vi "BenchA_v09_979.vi"() -> ()   [LabVIEW 2017]
uses:
  x64/Debug/BERTTA.dll
panel:
  out "element":bool
  out "Started:":string
  in  "SHUTDOWN":bool
  in  "MASTER CONTROL":bool
  in  "Tab Control":T1(tab)
  out "Output File":path caption="selected path"
  in  "Browse folder":path=path "" caption="start path"
  in  "Read Seq":bool
  in  "Save Seq":bool
  in  "Configuration file":path=path "C:/Users/shresplab/Desktop/BerttaConfiguration.lvm" caption="Filename"
  in  "OK Button 2":bool
  out "Boolean":bool
  in  "User (initials)":string
  in  "Project name":string
  in  "Description":string
  out "PUMP1":bool
  out "Target amount":dbl
  out "Scale weight":dbl
  out "Amount now":dbl
  out "Flow rate":dbl
  out "Time to target":dbl format="%<%H:%M:%S>t"
  out "Current step":dbl
  out "Target":dbl
  out "Amount now":dbl
  out "Amount now":dbl
  out "Target":dbl
  out "Current step":dbl
  out "Time to target":dbl format="%<%H:%M:%S>t"
  out "Flow rate":dbl
  out "Amount now":dbl
  out "Scale weight":dbl
  out "Target amount":dbl
  out "PUMP2":bool
  out "Sensor OK 6":bool
  out "Sensor OK 5":bool
  out "Sensor OK 4":bool
  out "Sensor OK 3":bool
  in  "OK Button":bool
  in  "Add comment":string
  out "PUMP3":bool
  out "Target amount":dbl
  out "Scale weight":dbl
  out "Amount now":dbl
  out "Flow rate":dbl
  out "Time to target":dbl format="%<%H:%M:%S>t"
  out "Current step":dbl
  out "Target":dbl
  out "Amount now":dbl
  out "Tr":dbl
  out "Tj in":dbl
  out "Tj out":dbl
  out "T set":dbl
  out "Current step":i32
  out "RPM":dbl
  out "Torque 2":dbl
  out "Waveform Chart 5":dynamicdata(graph)
  out "Waveform Chart 6":dynamicdata(graph)
  out "Waveform Chart 7":dynamicdata(graph)
  in  "Tab Control 2":T2(tab)
  out "Waveform Chart 3":dynamicdata(graph)
  out "Waveform Chart 8":dynamicdata(graph)
  out "Waveform Chart 11":dynamicdata(graph)
  out "Waveform Chart 13":dynamicdata(graph)
  out "Waveform Chart 9":dynamicdata(graph)
  out "Table":string[][](table)=[["14.8.2017 18.06.59", "0,000000", "417,670000", "-0,150000", "1,000000", "22,220000", "23,366837", "23,574959", "23,985852", "23,690000", "240,000000", "4,000000", "0,000000", "397,000000", "-397,000000", "1,000000"], ["14.8.2017 18.07.06", "0,000000", "417,640000", "-0,120000", "1,000000", "22,220000", "23,763115", "23,906257", "23,985694", "23,680000", "240,000000", "4,000000", "0,000000", "397,000000", "-397,000000", "1,000000"], ["14.8.2017 18.07.13", "0,000000", "417,640000", "-0,120000", "1,000000", "22,220000", "23,965922", "24,013440", "23,984906", "23,670000", "240,000000", "4,100000", "3,000000", "397,000000", "-397,000000", "1,000000"], ["14.8.2017 18.07.21", "0,000000", "417,640000", "-0,120000", "1,000000", "22,220000", "23,943860", "23,900110", "23,987113", "23,670000", "240,000000", "4,000000", "0,000000", "397,000000", "-397,000000", "1,000000"], ["14.8.2017 18.07.28", "0,000000", "417,640000", "-0,120000", "1,000000", "22,220000", "23,736328", "23,600018", "23,989004", "23,660000", "240,000000", "4,000000", "0,000000", "397,000000", "-397,000000", "1,000000"], ["14.8.2017 18.07.36", "0,000000", "417,640000", "-0,120000", "1,000000", "22,220000", "23,480910", "23,324538", "23,991053", "23,660000", "240,000000", "4,000000", "0,000000", "397,000000", "-397,000000", "1,000000"], ["14.8.2017 18.07.43", "0,000000", "417,640000", "-0,120000", "2,000000", "22,220000", "23,195579", "23,008270", "23,999093", "23,650000", "240,000000", "4,000000", "0,000000", "397,000000", "-397,000000", "1,000000"], ["14.8.2017 18.07.51", "0,000000", "417,650000", "-417,650000", "1,000000", "22,220000", "22,862541", "22,649021", "24,003979", "23,650000", "240,000000", "4,000000", "0,000000", "397,000000", "-397,000000", "2,000000"], ["14.8.2017 18.07.58", "0,000000", "417,640000", "0,010000", "1,000000", "22,220000", "22,541353", "22,354878", "24,005398", "23,650000", "240,000000", "4,000000", "0,000000", "397,000000", "-397,000000", "1,000000"], ["14.8.2017 18.08.06", "0,000000", "417,640000", "0,010000", "1,000000", "22,220000", "22,347931", "22,253738", "24,007605", "23,640000", "240,000000", "4,100000", "0,000000", "397,000000", "-397,000000", "1,000000"], ["14.8.2017 18.08.13", "0,000000", "417,640000", "0,010000", "1,000000", "22,220000", "22,329030", "22,302102", "24,006028", "23,640000", "240,000000", "4,000000", "0,000000", "395,820000", "-395,820000", "1,000000"], ["14.8.2017 18.08.20", "0,000000", "417,640000", "0,010000", "1,000000", "22,220000", "22,466849", "22,511320", "24,002403", "23,630000", "240,000000", "4,000000", "0,000000", "395,830000", "-0,010000", "1,000000"], ["14.8.2017 18.08.28", "0,000000", "417,640000", "0,010000", "1,000000", "22,220000", "22,707062", "22,835101", "24,000984", "23,620000", "240,000000", "4,000000", "0,000000", "395,830000", "-0,010000", "1,000000"], ["14.8.2017 18.08.35", "0,000000", "417,640000", "0,010000", "1,000000", "22,220000", "23,054104", "23,232979", "24,001299", "23,600000", "240,000000", "4,000000", "0,000000", "395,830000", "-0,010000", "1,000000"], ["14.8.2017 18.08.43", "0,000000", "417,640000", "0,010000", "1,000000", "22,220000", "23,412371", "23,522793", "24,002560", "23,590000", "240,000000", "4,000000", "0,000000", "395,820000", "0,000000", "1,000000"], ["14.8.2017 18.08.51", "0,000000", "417,640000", "0,010000", "1,000000", "22,220000", "23,596247", "23,656125", "24,003821", "23,580000", "240,000000", "4,000000", "0,000000", "395,820000", "0,000000", "1,000000"]]
  out "Boolean 4":bool
  out "Boolean 3":bool
  out "Boolean 2":bool
  in  "Reset 6":bool
  in  "Manual/Ramp":bool=TRUE
  in  "Array":dbl[][](array[numeric])=[[20.0, 0.0], [20.0, 0.0], [20.0, 0.0]]
  in  "?":bool
  in  "Time":dbl format="Time to target (min):                %#_g"
  out "Current temp":dbl format="Current temperature (S1):   %#_6g"
  in  "OK Button 3":bool
  in  "T ext / T ext 2":enum32{"Sensor 1", "Sensor 2"}(radio)
  out "Sensor OK":bool
  in  "T fail":dbl=20.0 format="Failsafe temperature:              %#_g"
  in  "Setpoint":dbl=20.0 format="Temperature target:                %#_6g"
  in  "Manual select":T3(radio)
  out "Waveform Chart":dynamicdata(graph)
  out "T external 2":dbl format="Current temperature (S2):    %#_g"
  in  "UPDATE TEMP":bool
  out "Led11 5":bool
  out "RPM":dbl format="%_4f"
  out "Led10 3":bool
  out "Led9 3":bool
  out "Led8 3":bool
  out "Led7 3":bool
  out "Led6 3":bool
  out "Led5 3":bool
  out "Led4 3":bool
  out "Led3 3":bool
  out "Led2 3":bool
  out "Led1 3":bool
  in  "PumpSeq 4":dbl[][](array[numeric])=[[0.0, 0.0, 0.0, 0.0, 0.0, 0.0, 0.0, 0.0, 0.0, 0.0], [0.0, 0.0, 0.0, 0.0, 0.0, 0.0, 0.0, 0.0, 0.0, 0.0], [0.0, 0.0, 0.0, 0.0, 0.0, 0.0, 0.0, 0.0, 0.0, 0.0], [0.0, 0.0, 0.0, 0.0, 0.0, 0.0, 0.0, 0.0, 0.0, 0.0], [0.0, 0.0, 0.0, 0.0, 0.0, 0.0, 0.0, 0.0, 0.0, 0.0], [0.0, 0.0, 0.0, 0.0, 0.0, 0.0, 0.0, 0.0, 0.0, 0.0], [0.0, 0.0, 0.0, 0.0, 0.0, 0.0, 0.0, 0.0, 0.0, 0.0], [0.0, 0.0, 0.0, 0.0, 0.0, 0.0, 0.0, 0.0, 0.0, 0.0], [0.0, 0.0, 0.0, 0.0, 0.0, 0.0, 0.0, 0.0, 0.0, 0.0], [0.0, 0.0, 0.0, 0.0, 0.0, 0.0, 0.0, 0.0, 0.0, 0.0]]
  in  "?":bool
  out "Flow rate (g/min)":dbl
  out "Scale reading":dbl
  out "Step amount now":dbl
  in  "Grams / min":dbl
  out "Waveform Chart 14":dynamicdata(graph)
  in  "?":bool
  out "Total amount now":dbl
  out "Led11 4":bool
  in  "Reset 5":bool
  out "Elapsed / step":i32
  out "Time to target":dbl format="%<%H:%M:%S>t"
  in  "OK Button 4":bool
  out "Led11":bool
  out "RPM":dbl format="%_4f"
  out "Led10":bool
  out "Led9":bool
  out "Led8":bool
  out "Led7":bool
  out "Led6":bool
  out "Led5":bool
  out "Led4":bool
  out "Led3":bool
  out "Led2":bool
  out "Led1":bool
  in  "PumpSeq 2":dbl[][](array[numeric])=[[0.0, 0.0, 0.0, 0.0, 0.0, 0.0, 0.0, 0.0, 0.0, 0.0], [0.0, 0.0, 0.0, 0.0, 0.0, 0.0, 0.0, 0.0, 0.0, 0.0], [0.0, 0.0, 0.0, 0.0, 0.0, 0.0, 0.0, 0.0, 0.0, 0.0], [0.0, 0.0, 0.0, 0.0, 0.0, 0.0, 0.0, 0.0, 0.0, 0.0], [0.0, 0.0, 0.0, 0.0, 0.0, 0.0, 0.0, 0.0, 0.0, 0.0], [0.0, 0.0, 0.0, 0.0, 0.0, 0.0, 0.0, 0.0, 0.0, 0.0], [0.0, 0.0, 0.0, 0.0, 0.0, 0.0, 0.0, 0.0, 0.0, 0.0], [0.0, 0.0, 0.0, 0.0, 0.0, 0.0, 0.0, 0.0, 0.0, 0.0], [0.0, 0.0, 0.0, 0.0, 0.0, 0.0, 0.0, 0.0, 0.0, 0.0], [0.0, 0.0, 0.0, 0.0, 0.0, 0.0, 0.0, 0.0, 0.0, 0.0]]
  in  "?":bool
  out "Flow rate (g/min)":dbl
  out "Scale reading":dbl
  out "Step amount now":dbl
  in  "Grams / min":dbl
  out "Waveform Chart 10":dynamicdata(graph)
  in  "?":bool
  out "Total amount now":dbl
  out "Led11":bool
  in  "Reset 3":bool
  out "Elapsed / step":i32
  out "Time to target":dbl format="%<%H:%M:%S>t"
  in  "OK Button 5":bool
  out "Led11 3":bool
  out "RPM":dbl format="%_4f"
  out "Led10 2":bool
  out "Led9 2":bool
  out "Led8 2":bool
  out "Led7 2":bool
  out "Led6 2":bool
  out "Led5 2":bool
  out "Led4 2":bool
  out "Led3 2":bool
  out "Led2 2":bool
  out "Led1 2":bool
  in  "PumpSeq 3":dbl[][](array[numeric])=[[0.0, 0.0, 0.0, 0.0, 0.0, 0.0, 0.0, 0.0, 0.0, 0.0], [0.0, 0.0, 0.0, 0.0, 0.0, 0.0, 0.0, 0.0, 0.0, 0.0], [0.0, 0.0, 0.0, 0.0, 0.0, 0.0, 0.0, 0.0, 0.0, 0.0], [0.0, 0.0, 0.0, 0.0, 0.0, 0.0, 0.0, 0.0, 0.0, 0.0], [0.0, 0.0, 0.0, 0.0, 0.0, 0.0, 0.0, 0.0, 0.0, 0.0], [0.0, 0.0, 0.0, 0.0, 0.0, 0.0, 0.0, 0.0, 0.0, 0.0], [0.0, 0.0, 0.0, 0.0, 0.0, 0.0, 0.0, 0.0, 0.0, 0.0], [0.0, 0.0, 0.0, 0.0, 0.0, 0.0, 0.0, 0.0, 0.0, 0.0], [0.0, 0.0, 0.0, 0.0, 0.0, 0.0, 0.0, 0.0, 0.0, 0.0], [0.0, 0.0, 0.0, 0.0, 0.0, 0.0, 0.0, 0.0, 0.0, 0.0]]
  in  "?":bool
  out "Flow rate (g/min)":dbl
  out "Scale reading":dbl
  out "Step amount now":dbl
  in  "Grams / min":dbl
  out "Waveform Chart 12":dynamicdata(graph)
  in  "?":bool
  out "Total amount now":dbl
  out "Led11 2":bool
  in  "Reset 4":bool
  out "Elapsed / step":i32
  out "Time to target":dbl format="%<%H:%M:%S>t"
  in  "OK Button 6":bool
  out "Waveform Chart 15":dynamicdata(graph)
  in  "?":bool
  in  "OK Button 8":bool
  in  "PORT":i32=6
  in  "Remote / Manual":bool
  in  "Set RPM":i32
  out "RPM":dbl
  out "Torque":dbl
  out "Waveform Chart 4":dynamicdata(graph)
  in  "OK Button 7":bool
  out "PortDev out":dbl[](array[numeric])
  in  "Save PortDev":bool
  out "PortDev in":dbl[](array[numeric])
  in  "dev1":i32
  in  "dev2":i32
  in  "dev3":i32
  in  "dev4":i32
  in  "dev5":i32
  in  "dev6":i32
  in  "dev8":i32
  in  "port1":i32
  in  "port2":i32
  in  "port3":i32
  in  "port4":i32
  in  "port5":i32
  in  "port6":i32
  in  "port7":i32
  in  "port8":i32
  in  "dev7":i32
  in  "Treshold (T/C)":dbl=0.5
  out "DAQ 9217 (PT100)":errorcluster
  out "Config File":dbl[][](array[numeric])
  in  "device name (PAM)":tag="cDAQ9188XT-1C3BF12Mod7"
  # "Temperature sensor:"
  # "Manual control:"
  # "PUMP & SCALE 1"
  # "STEP"
  # "TOTAL"
  # "PUMP & SCALE 2"
  # "STEP"
  # "TOTAL"
  # "PUMP & SCALE 3"
  # "STEP"
  # "TOTAL"
  # "Temperature control parameter"
  # "Secondary temperature sensor"
  # "Temp target"
  # "Time target"
  # "Grams    /   min"
  # "End of sequence"
  # "Manual control"
  # "Grams    /   min"
  # "End of sequence"
  # "Manual control"
  # "Grams    /   min"
  # "End of sequence"
  # "Manual control"
  # "PAM control"
  # "dev1 and dev2 always to port1 and 2\nport1 = port2 = Lauda\n\ndev3 and dev4 always to port3 and port4\nport3 = port4 = Heidolph"
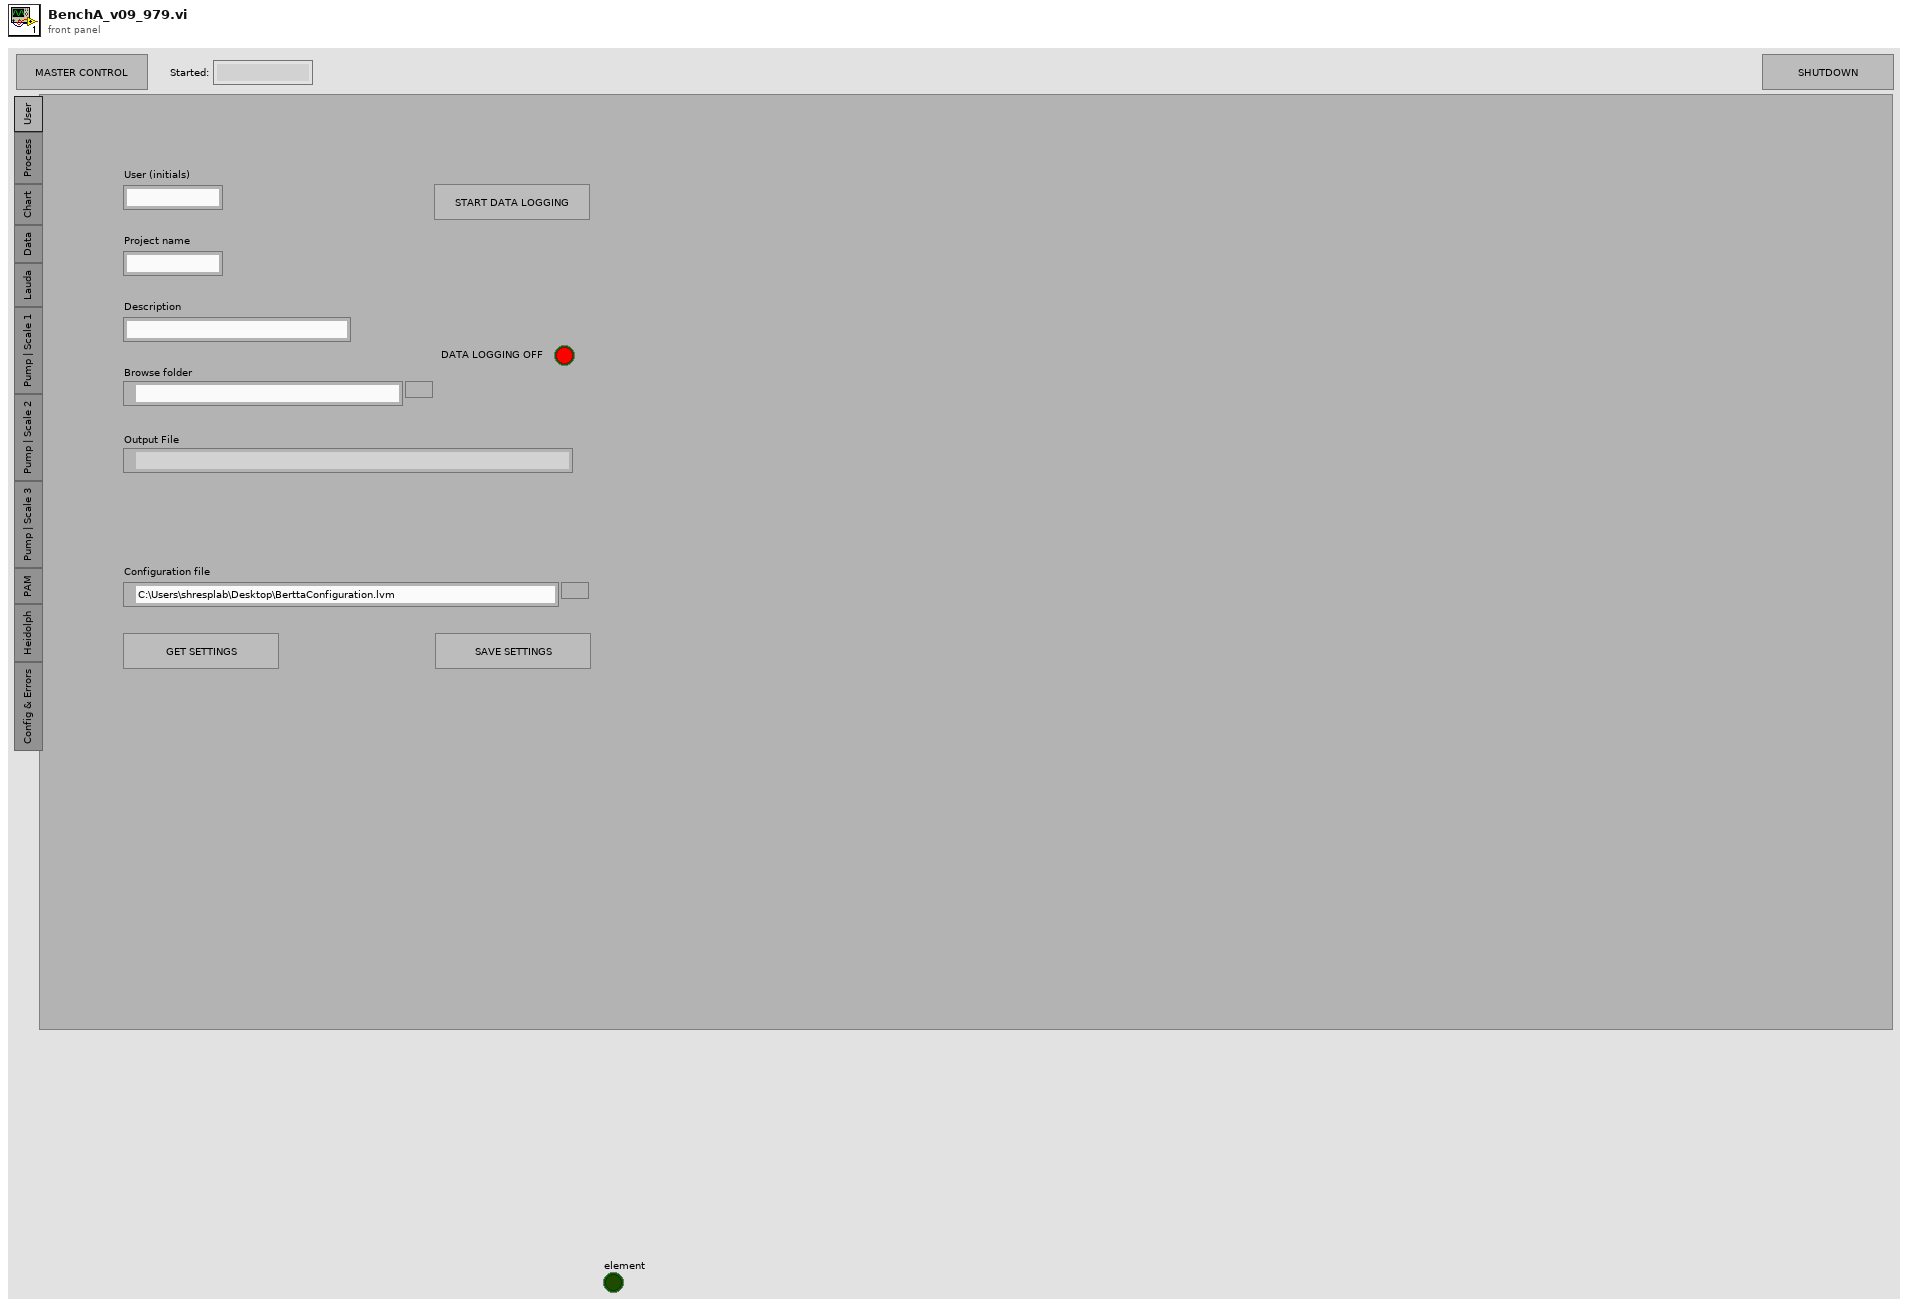
[diagram p1: front panel]
types:
  T1 = enum32{"User", "Process", "Chart", "Data", "Lauda", "Pump | Scale 1", "Pump | Scale 2", "Pump | Scale 3", "PAM", "Heidolph", "Config & Errors"}
  T2 = enum32{"Temperatures", "Scale / Pump 1", "Scale / Pump 2", "Scale / Pump 3", "RPM / torque"}
  T3 = enum32{"Reactor temperature", "Jacket temperature"}
diagram:
  n1 = while {
    i -> [w62]
    stop <- FALSE stop-if-true
    w48 = 0.0 ("y")
    # "PAM Control"
    # "Muutettava\nlaudan kutsun \nosalta"
    # "SCALE & PUMP 1"
    # "SCALE & PUMP 3"
    # "SCALE & PUMP 2"
    n2 = Not(x="MASTER CONTROL") -> (.not. x?=w287:bool)
    n3 = Boolean To (0,1)(Boolean=w287) -> (0, 1=w288:i16)
    n4 = Not(x="Manual/Ramp") -> (.not. x?=w55:bool)
    n5 = for {
      N: w288 -> [_]
      n6 = Get Date/Time String(want seconds? (F)=TRUE) -> (time string=→"Started:":string)  [unwired: 2 in, 1 out]
    }
    n7 = Boolean To (0,1)(Boolean=w55) -> (0, 1=w37:i16)
    n8 = feedback #1() -> (w43:bool)  [unwired: 1 in]
    n9 = feedback-in #1("Manual/Ramp") -> ()
    n10 = Not Equal?(x=w43, y="Manual/Ramp") -> (x != y?=w40:bool)
    n11 = Boolean To (0,1)(Boolean="SHUTDOWN") -> (0, 1=w272:i16)
    n12 = for {
      N: w272 -> [_]
      tunnel: [w404] -> w286 mode=indexing
      i -> [w406]
      n13 = control-ref of="This VI"() -> (w409:refnum<vi>)
      n14 = invoke class="VI" method="Default Vals.Reinit All"(reference=w409) -> (reference out=w407:refnum<vi>, error out=w408:errorcluster)  [unwired: 2 in, 1 out]
      n15 = Greater?(x=w406, y=0) -> (0:w404:bool)
      n16 = Close Reference(reference=w407, error in (no error)=w408) -> ()  [unwired: 1 out]
    }
    n17 = feedback #2() -> (w35:bool)  [unwired: 1 in]
    n18 = call "MReadRS232_2.vi"("port1"="port1", "dev1"="dev1", "port2"="port2", "dev2"="dev2", "port3"="port3", "dev7"="dev7", "dev8"="dev8", "port7"="port7", "port8"="port8", "dev5"="dev5", "port5"="port5", "dev4"="dev4", "dev6"="dev6", "port6"="port6", "port4"="port4", "dev3"="dev3") -> ("output array"=w66:dbl[], "params"=w10:dbl[])  [unwired: 2 in]
    "PortDev in" <- w66
    n19 = feedback #3(0) -> (w270:i32)
    n20 = formula code="out = 0;\nint out2=0;\nif(in==1 ) out2 = 1;\nif(in2==1) out = 1;"("in"=w272, "in2"=w270) -> ("out"=w274:dbl, "out2"=w271:i32)
    n21 = feedback-in #3(w271) -> ()
    n22 = And(x="MASTER CONTROL", y=w35) -> (x .and. y?=w93:bool)
    n23 = feedback #4() -> (w84:bool)  [unwired: 1 in]
    n24 = feedback-in #4("MASTER CONTROL") -> ()
    n25 = Boolean To (0,1)(Boolean=w93) -> (0, 1=w82:i16)
    n26 = Not Equal?(x=w84, y="MASTER CONTROL") -> (x != y?=w83:bool)
    n27 = Boolean To (0,1)(Boolean=w83) -> (0, 1=w81:i16)
    n28 = Equal?(x=w274, y=1.0) -> (x = y?=w273:bool)
    n29 = Index Array(array=w286, index=0) -> (element=→"element":bool)
    n30 = Or(x=w81, y=w82) -> (x .or. y?=w80:i16)
    n31 = for {
      N: w80 -> [_]
      tunnel: "Time" -> [w356]
      shift-right: [w355] -> w94
      shift-left: _ -> [_]
      tunnel: "Setpoint" -> [w353]
      shift-right: [w352] -> w91
      shift-left: _ -> [_]
      n32 = Add(x=w353, y=0.0) -> (x+y=w352:dbl)
      n33 = Add(x=w356, y=0.0) -> (x+y=w355:dbl)
    }
    n34 = Stop(stop? (T)=w273) -> ()
    n35 = Boolean To (0,1)(Boolean="Save PortDev") -> (0, 1=w65:i16)
    n36 = feedback-in #5(w91) -> ()
    n37 = feedback #5() -> (w92:dbl)  [unwired: 1 in]
    n38 = for {
      N: w65 -> [_]
      tunnel: w66 -> [w351]
      tunnel: "Save PortDev" -> [w349]
      n39 = call "Convert to Dynamic Data"("Array"=w351) -> ("Dynamic Data Type"=w350:dynamicdata)  [unwired: 3 in]
      n40 = call "Write To Measurement File3"("Signals"=w350, "Reset"=w349) -> ()  [unwired: 15 in, 3 out]
    }
    n41 = Not(x="?") -> (.not. x?=w87:bool)
    n42 = Not Equal?(x=w92, y=w91) -> (x != y?=w90:bool)
    n43 = Boolean To (0,1)(Boolean=w87) -> (0, 1=w89:i16)
    n44 = Boolean To (0,1)(Boolean=w90) -> (0, 1=w85:i16)
    n45 = Boolean To (0,1)(Boolean="MASTER CONTROL") -> (0, 1=w86:i16)
    n46 = feedback-in #6("Remote / Manual") -> ()
    n47 = feedback #6() -> (w32:bool)  [unwired: 1 in]
    n48 = Boolean To (0,1)(Boolean="Remote / Manual") -> (0, 1=w30:i16)
    n49 = call "ramp_simple_1.vi"("pause"=w89, "time_set"=w94, "array"=w10, "reset"=w85, "port"="port1", "master"=w86, "T_sp"=w91, "treshold"="Treshold (T/C)") -> ("Tin"=w97:dbl, "Tr"=w98:dbl, "target_reached"=w53:dbl, "T control"=w17:dbl)  [unwired: 3 in, 1 out]
    "Tr" <- w98
    "Current temp" <- w98
    n50 = for {
      N: w37 -> [_]
      tunnel: w53 -> [w308]
      tunnel: [w298] -> w41
      tunnel: "Reset 6" -> [w300]
      tunnel: [w301] -> w44
      n51 = feedback #7() -> (w302:i32)  [unwired: 1 in]
      n52 = Boolean To (0,1)(Boolean=w300) -> (0, 1=w303:i16)
      n53 = call "count_rising_edge.vi"("reset"=w303, "target_reached"=w308) -> ("element 2"=w301:i32)  [unwired: 9 in]
      n54 = feedback-in #7(w301) -> ()
      n55 = Not Equal?(x=w302, y=w301) -> (x != y?=w299:bool)
      n56 = Or(x=w300, y=w299) -> (x .or. y?=w298:bool)
      n57 = Index Array(array="Array", index (row)=w301, index (col)=1 ("disabled index (col)")) -> (element=w304:dbl)
      n58 = Index Array(array="Array", index (row)=w301, index (col)=0 ("disabled index (col)")) -> (element=w305:dbl)
      n59 = property on="Time" class="DigNum (strict)"("Val(Sgnl)"=w304) -> ()  [unwired: 2 in, 2 out]
      n60 = property on="Setpoint" class="DigNum (strict)"("Val(Sgnl)"=w305) -> ()  [unwired: 2 in, 2 out]
    }
    n61 = Or(x=w40, y=w41) -> (x .or. y?=w39:bool)
    n62 = Or(x="UPDATE TEMP", y=w39) -> (x .or. y?=w36:bool)
    n63 = feedback-in #2(w36) -> ()
    n64 = formula code="LED0=0;\nLED1=0;\nLED2=0;\nLED3=0;\nif(step==0 && man==1) LED0=1;\nif(step==1 && man==1) LED1=1;\nif(step==2 && man==1) LED2=1;\nif(step==3 && man==1) LED3=1;"("step"=w44, "man"=w37) -> ("LED0"=w52:dbl, "LED1"=w51:dbl, "LED2"=w50:dbl, "LED3"=w49:dbl)
    n65 = Not Equal?(x=w52, y=w48) -> (x != y?=→"Boolean 2":bool)
    n66 = Not Equal?(x=w51, y=w48) -> (x != y?=→"Boolean 3":bool)
    n67 = Not Equal?(x=w50, y=w48) -> (x != y?=→"Boolean 4":bool)
    n68 = Not Equal?(x=w49, y=w48) -> ()  [unwired: 1 out]
    n69 = Less?(x=w62, y=1.0) -> (x < y?=w60:bool)
    n70 = Not Equal?(x=w32, y="Remote / Manual") -> (x != y?=w31:bool)
    n71 = Boolean To (0,1)(Boolean=w31) -> (0, 1=w33:i16)
    n72 = for {
      N: w33 -> [_]
      tunnel: "port3" -> [w296]
      n73 = dll-call lib="C:/Users/shresplab/OneDrive - Kemira Oyj/Documents/GitHub/Bertta/BERTTA/x64/Debug/BERTTA.dll" fn="hei_query"("port"=w296, "q"=5) -> ()  [unwired: 6 in, 2 out]
    }
    n74 = Index Array(array=w10, index=3) -> (element=w25:dbl)
    "RPM" <- w25
    "RPM" <- w25
    n75 = Index Array(array=w10, index=2) -> (element=w27:dbl)
    n76 = Boolean To (0,1)(Boolean=w60) -> (0, 1=w61:i16)
    n77 = Divide(x=w27, y=10.0) -> (x/y=w24:dbl)
    "Torque" <- w24
    "Torque 2" <- w24
    n78 = for {
      N: w30 -> [_]
      tunnel: "port3" -> [w294]
      n79 = dll-call lib="C:/Users/shresplab/OneDrive - Kemira Oyj/Documents/GitHub/Bertta/BERTTA/x64/Debug/BERTTA.dll" fn="heidolph"("port"=w294, "speed"="Set RPM") -> ()  [unwired: 6 in, 2 out]
    }
    n80 = for {
      N: w61 -> [_]
      tunnel: w60 -> [w344]
      n81 = while {
        tunnel: [w347] -> w343
        tunnel: w344 -> [w345]
        stop <- w348 stop-if-true
        n82 = call "Read From Measurement File2"("Enable"=TRUE, "Reset"=w345) -> ("Signals"=w347:dynamicdata, "EOF?"=w348:bool)  [unwired: 4 in, 4 out]
      }
      n83 = call "Convert from Dynamic Data2"("Dynamic Data Type"=w343) -> ("Array"=w326:dbl[])  [unwired: 3 in]
      "PortDev out" <- w326
      n84 = Index Array(array=w326, index=6) -> (element=w319:dbl)
      n85 = Index Array(array=w326, index=7) -> (element=w318:dbl)
      n86 = Index Array(array=w326, index=5) -> (element=w320:dbl)
      n87 = Index Array(array=w326, index=4) -> (element=w321:dbl)
      n88 = Index Array(array=w326, index=0) -> (element=w325:dbl)
      n89 = Index Array(array=w326, index=1) -> (element=w324:dbl)
      n90 = Index Array(array=w326, index=3) -> (element=w322:dbl)
      n91 = Index Array(array=w326, index=2) -> (element=w323:dbl)
      n92 = property on="dev4" class="DigNum (strict)"("Val(Sgnl)"=w318) -> ()  [unwired: 2 in, 2 out]
      n93 = property on="dev3" class="DigNum (strict)"("Val(Sgnl)"=w320) -> ()  [unwired: 2 in, 2 out]
      n94 = property on="port4" class="DigNum (strict)"("Val(Sgnl)"=w319) -> ()  [unwired: 2 in, 2 out]
      n95 = property on="port1" class="DigNum (strict)"("Val(Sgnl)"=w325) -> ()  [unwired: 2 in, 2 out]
      n96 = property on="dev1" class="DigNum (strict)"("Val(Sgnl)"=w324) -> ()  [unwired: 2 in, 2 out]
      n97 = property on="port2" class="DigNum (strict)"("Val(Sgnl)"=w323) -> ()  [unwired: 2 in, 2 out]
      n98 = property on="dev2" class="DigNum (strict)"("Val(Sgnl)"=w322) -> ()  [unwired: 2 in, 2 out]
      n99 = property on="port3" class="DigNum (strict)"("Val(Sgnl)"=w321) -> ()  [unwired: 2 in, 2 out]
      n100 = Index Array(array=w326, index=14) -> (element=w311:dbl)
      n101 = Index Array(array=w326, index=15) -> (element=w310:dbl)
      n102 = Index Array(array=w326, index=13) -> (element=w312:dbl)
      n103 = Index Array(array=w326, index=12) -> (element=w313:dbl)
      n104 = Index Array(array=w326, index=8) -> (element=w317:dbl)
      n105 = Index Array(array=w326, index=9) -> (element=w316:dbl)
      n106 = Index Array(array=w326, index=11) -> (element=w314:dbl)
      n107 = Index Array(array=w326, index=10) -> (element=w315:dbl)
      n108 = property on="port5" class="DigNum (strict)"("Val(Sgnl)"=w317) -> ()  [unwired: 2 in, 2 out]
      n109 = property on="dev5" class="DigNum (strict)"("Val(Sgnl)"=w316) -> ()  [unwired: 2 in, 2 out]
      n110 = property on="port6" class="DigNum (strict)"("Val(Sgnl)"=w315) -> ()  [unwired: 2 in, 2 out]
      n111 = property on="dev6" class="DigNum (strict)"("Val(Sgnl)"=w314) -> ()  [unwired: 2 in, 2 out]
      n112 = property on="port7" class="DigNum (strict)"("Val(Sgnl)"=w313) -> ()  [unwired: 2 in, 2 out]
      n113 = property on="dev7" class="DigNum (strict)"("Val(Sgnl)"=w312) -> ()  [unwired: 2 in, 2 out]
      n114 = property on="port8" class="DigNum (strict)"("Val(Sgnl)"=w311) -> ()  [unwired: 2 in, 2 out]
      n115 = property on="dev8" class="DigNum (strict)"("Val(Sgnl)"=w310) -> ()  [unwired: 2 in, 2 out]
    }
    n116 = Merge Signals(w25, w24) -> (w23:dynamicdata)
    "Waveform Chart 4" <- w23
    "Waveform Chart 6" <- w23
    "Waveform Chart 9" <- w23
    n117 = call "LaudaLedCtrl.vi"("Manual select"="Manual select", "T ext / T ext in"="T ext / T ext 2", "Lauda port"="port1") -> ("Sensor OK 5"=→"Sensor OK 5":bool, "Sensor OK 3"=→"Sensor OK 3":bool, "Sensor OK 4"=→"Sensor OK 4":bool, "Sensor OK 6"=→"Sensor OK 6":bool)  [unwired: 5 in]
    n118 = call "LaudaDAQ.vi"() -> ("error out"=→"DAQ 9217 (PT100)":errorcluster, 1:"Tj out"=→"Tj out":dbl, "data"=w162:dynamicdata, "Sensor OK"=→"Sensor OK":bool, 4:"Tj out"=→"Tj in":dbl, "T external 2"=→"T external 2":dbl)  [unwired: 6 in]
    n119 = Boolean To (0,1)(Boolean="OK Button 3") -> (0, 1=w109:i16)
    n120 = for {
      N: w109 -> [_]
      n121 = property on="Waveform Chart" class="WFChart (strict)"("History Data"=dynamicdata[] []) -> ()  [unwired: 2 in, 2 out]
    }
    n122 = Merge Signals(w17, w98, w97, w162) -> (w163:dynamicdata)
    "Waveform Chart 3" <- w163
    "Waveform Chart" <- w163
    "Waveform Chart 5" <- w163
    n123 = Boolean To (0,1)(Boolean="OK Button 4") -> (0, 1=w107:i16)
    n124 = for {
      N: w107 -> [_]
      n125 = property on="Waveform Chart 14" class="WFChart (strict)"("History Data"=dynamicdata[] []) -> ()  [unwired: 2 in, 2 out]
    }
    n126 = Boolean To (0,1)(Boolean="?") -> (0, 1=w171:i16)
    n127 = Boolean To (0,1)(Boolean="?") -> (0, 1=w175:i16)
    n128 = Boolean To (0,1)(Boolean="MASTER CONTROL") -> (0, 1=w167:i16)
    n129 = Boolean To (0,1)(Boolean="Reset 5") -> (0, 1=w174:i16)
    n130 = Boolean To (0,1)(Boolean="OK Button 5") -> (0, 1=w105:i16)
    n131 = Index Array(array="PumpSeq 4", index (col)=0) -> (element=w179:dbl[])  [unwired: 1 in]
    n132 = Index Array(array="PumpSeq 4", index (col)=1) -> (element=w200:dbl[])  [unwired: 1 in]
    n133 = for {
      N: w105 -> [_]
      n134 = property on="Waveform Chart 10" class="WFChart (strict)"("History Data"=dynamicdata[] []) -> ()  [unwired: 2 in, 2 out]
    }
    n135 = call "pumpsec_09_P1.vi"("reset"=w174, "master"=w167, "manual"=w171, "pause"=w175, "Array"=w10, "Target"=w179, "fr_manual"="Grams / min", "Time"=w200) -> ("pumpCtrl"=w146:dbl, "totaltarget"=→"Target":dbl, "target_step"=→"Target amount":dbl, "REGLO D"=w21:dbl, "time_to_target"=→"Time to target" →"Time to target":dbl, "step_fr"=w123:dbl, "amount_step"=→"Amount now" →"Step amount now":dbl, "Scale"=w158:dbl, "elapsed_step"=→"Elapsed / step":dbl, "params"=w197:dbl[])  [unwired: 8 in, 2 out]
    "Flow rate" <- w123
    "Scale weight" <- w158
    "Scale reading" <- w158
    "Flow rate (g/min)" <- w123
    "RPM" <- w21
    n136 = Greater?(x=w146, y=70.0) -> (0:→"PUMP1":bool)
    n137 = Merge Signals(w158, w123) -> (w166:dynamicdata)
    "Waveform Chart 8" <- w166
    "Waveform Chart 14" <- w166
    n138 = Index Array(array=w197, index=1) -> (element=w194:dbl)
    n139 = Index Array(array=w197, index=2) -> (element=→"Amount now" →"Total amount now":dbl)
    n140 = Add(x=1.0, y=w194) -> (x+y=w124:dbl)
    "Current step" <- w124
    n141 = Boolean To (0,1)(Boolean="OK Button 6") -> (0, 1=w103:i16)
    n142 = for {
      N: w103 -> [_]
      n143 = property on="Waveform Chart 12" class="WFChart (strict)"("History Data"=dynamicdata[] []) -> ()  [unwired: 2 in, 2 out]
    }
    n144 = call "STEPINDICATOR_091_2.vi"("current step"=w124, "enable"=i16 1, "manual"=w171) -> ("Led 8"=→"Led8 3":bool, "Led 10"=→"Led10 3":bool, "Led 11"=→"Led11 4":bool, "Led 7"=→"Led7 3":bool, "Led 1"=→"Led1 3":bool, "Led 6"=→"Led6 3":bool, "Led 2"=→"Led2 3":bool, "Led 12"=→"Led11 5":bool, "Led 5"=→"Led5 3":bool, "Led 4"=→"Led4 3":bool, "Led 3"=→"Led3 3":bool, "Led 9"=→"Led9 3":bool)  [unwired: 1 in]
    n145 = Boolean To (0,1)(Boolean="OK Button 7") -> (0, 1=w101:i16)
    n146 = for {
      N: w101 -> [_]
      n147 = property on="Waveform Chart 4" class="WFChart (strict)"("History Data"=dynamicdata[] []) -> ()  [unwired: 2 in, 2 out]
    }
    n148 = Boolean To (0,1)(Boolean="OK Button 8") -> (0, 1=w4:i16)
    n149 = for {
      N: w4 -> [_]
      n150 = property on="Waveform Chart 15" class="WFChart (strict)"("History Data"=dynamicdata[] []) -> ()  [unwired: 2 in, 2 out]
    }
    n151 = Boolean To (0,1)(Boolean="?") -> (0, 1=w234:i16)
    n152 = Boolean To (0,1)(Boolean="?") -> (0, 1=w261:i16)
    n153 = Boolean To (0,1)(Boolean="Reset 3") -> (0, 1=w259:i16)
    n154 = Boolean To (0,1)(Boolean="MASTER CONTROL") -> (0, 1=w253:i16)
    n155 = Index Array(array="PumpSeq 2", index (col)=0 ("disabled index (col)")) -> (element=w264:dbl[])  [unwired: 1 in]
    n156 = Index Array(array="PumpSeq 2", index (col)=1 ("disabled index (col)")) -> (element=w263:dbl[])  [unwired: 1 in]
    n157 = call "pumpsec_09_P2.vi"("reset"=w259, "master"=w253, "manual"=w234, "pause"=w261, "Array"=w10, "Target"=w264, "fr_manual"="Grams / min", "Time"=w263) -> ("pumpCtrl"=w142:dbl, "totaltarget"=→"Target":dbl, "target_step"=→"Target amount":dbl, "REGLO D"=w20:dbl, "time_to_target"=→"Time to target" →"Time to target":dbl, "step_fr"=w161:dbl, "amount_step"=→"Amount now" →"Step amount now":dbl, "Scale"=w157:dbl, "elapsed_step"=→"Elapsed / step":dbl, "params"=w254:dbl[])  [unwired: 8 in, 2 out]
    "Scale weight" <- w157
    "Flow rate" <- w161
    "Scale reading" <- w157
    "Flow rate (g/min)" <- w161
    "RPM" <- w20
    n158 = Greater?(x=w142, y=70.0) -> (0:→"PUMP2":bool)
    n159 = Index Array(array=w254, index=1) -> (element=w257:dbl)
    n160 = Index Array(array=w254, index=2) -> (element=→"Amount now" →"Total amount now":dbl)
    n161 = Merge Signals(w157, w161) -> (w168:dynamicdata)
    "Waveform Chart 11" <- w168
    "Waveform Chart 10" <- w168
    n162 = Add(x=1.0, y=w257) -> (x+y=w251:dbl)
    "Current step" <- w251
    n163 = call "STEPINDICATOR_091_2.vi"("current step"=w251, "enable"=i16 1, "manual"=w234) -> ("Led 8"=→"Led8":bool, "Led 10"=→"Led10":bool, "Led 11"=→"Led11":bool, "Led 7"=→"Led7":bool, "Led 1"=→"Led1":bool, "Led 6"=→"Led6":bool, "Led 2"=→"Led2":bool, "Led 12"=→"Led11":bool, "Led 5"=→"Led5":bool, "Led 4"=→"Led4":bool, "Led 3"=→"Led3":bool, "Led 9"=→"Led9":bool)  [unwired: 1 in]
    n164 = Boolean To (0,1)(Boolean="?") -> (0, 1=w228:i16)
    n165 = Boolean To (0,1)(Boolean="?") -> (0, 1=w227:i16)
    n166 = Boolean To (0,1)(Boolean="MASTER CONTROL") -> (0, 1=w229:i16)
    n167 = Boolean To (0,1)(Boolean="Reset 4") -> (0, 1=w209:i16)
    n168 = Index Array(array="PumpSeq 3", index (col)=0 ("disabled index (col)")) -> (element=w212:dbl[])  [unwired: 1 in]
    n169 = Index Array(array="PumpSeq 3", index (col)=1 ("disabled index (col)")) -> (element=w211:dbl[])  [unwired: 1 in]
    n170 = dll-call lib="C:/Users/shresplab/OneDrive - Kemira Oyj/Documents/GitHub/Bertta/BERTTA/x64/Debug/BERTTA.dll" fn="lauda"("port"=1, "set_temp"=w17) -> ()  [unwired: 6 in, 2 out]
    n171 = call "pumpsec_09_P3.vi"("reset"=w209, "master"=w229, "manual"=w228, "pause"=w227, "Array"=w10, "Target"=w212, "fr_manual"="Grams / min", "Time"=w211) -> ("pumpCtrl"=w139:dbl, "totaltarget"=→"Target":dbl, "target_step"=→"Target amount":dbl, "REGLO D"=w19:dbl, "time_to_target"=→"Time to target" →"Time to target":dbl, "step_fr"=w160:dbl, "amount_step"=→"Amount now" →"Step amount now":dbl, "Scale"=w156:dbl, "elapsed_step"=→"Elapsed / step":dbl, "params"=w202:dbl[])  [unwired: 8 in, 2 out]
    "Scale weight" <- w156
    "Flow rate" <- w160
    "Scale reading" <- w156
    "Flow rate (g/min)" <- w160
    "RPM" <- w19
    n172 = Greater?(x=w139, y=70.0) -> (0:→"PUMP3":bool)
    n173 = Merge Signals(w158, w157, w156) -> (→"Waveform Chart 7":dynamicdata)
    n174 = Index Array(array=w202, index=1) -> (element=w203:dbl)
    n175 = Index Array(array=w202, index=2) -> (element=→"Amount now" →"Total amount now":dbl)
    n176 = Add(x=1.0, y=w203) -> (x+y=w201:dbl)
    "Current step" <- w201
    n177 = call "Convert to Dynamic Data4"("2D Array"="PumpSeq 3") -> ("Dynamic Data Type"=w115:dynamicdata)  [unwired: 3 in]
    n178 = call "Convert to Dynamic Data3"("2D Array"="PumpSeq 2") -> ("Dynamic Data Type"=w117:dynamicdata)  [unwired: 3 in]
    n179 = call "Convert to Dynamic Data2"("2D Array"="PumpSeq 4") -> ("Dynamic Data Type"=w120:dynamicdata)  [unwired: 3 in]
    n180 = call "RegloAnalog.vi"("REGLO D"=w19, "REGLO D 2"=w20, "REGLO D 3"=w21) -> ()  [unwired: 9 in]
    n181 = Merge Signals(w115, w117, w120) -> (w119:dynamicdata)
    n182 = Merge Signals(w156, w160) -> (w165:dynamicdata)
    "Waveform Chart 13" <- w165
    "Waveform Chart 12" <- w165
    n183 = Boolean To (0,1)(Boolean="Save Seq") -> (0, 1=w114:i16)
    n184 = for {
      N: w114 -> [_]
      tunnel: w119 -> [w402]
      tunnel: "Configuration file" -> [w403]
      tunnel: "Save Seq" -> [w401]
      n185 = call "Write To Measurement File2"("Signals"=w402, "Reset"=w401, "Filename"=w403) -> ()  [unwired: 14 in, 3 out]
    }
    n186 = call "STEPINDICATOR_091_4.vi"("current step"=w201, "enable"=i16 1, "manual"=w228) -> ("Led 8"=→"Led8 2":bool, "Led 10"=→"Led10 2":bool, "Led 11"=→"Led11 2":bool, "Led 7"=→"Led7 2":bool, "Led 1"=→"Led1 2":bool, "Led 6"=→"Led6 2":bool, "Led 2"=→"Led2 2":bool, "Led 12"=→"Led11 3":bool, "Led 5"=→"Led5 2":bool, "Led 4"=→"Led4 2":bool, "Led 3"=→"Led3 2":bool, "Led 9"=→"Led9 2":bool)  [unwired: 1 in]
    n187 = Merge Signals(w166, w168, w165) -> (w164:dynamicdata)
    n188 = Boolean To (0,1)(Boolean="Read Seq") -> (0, 1=w113:i16)
    n189 = for {
      N: w113 -> [_]
      tunnel: "Configuration file" -> [w374]
      tunnel: "Read Seq" -> [w373]
      n190 = while {
        tunnel: [w400] -> w396
        tunnel: w374 -> [w399]
        tunnel: w373 -> [w397]
        stop <- w398 stop-if-true
        n191 = call "Read From Measurement File"("Filename"=w399, "Reset"=w397) -> ("Signals"=w400:dynamicdata, "EOF?"=w398:bool)  [unwired: 4 in, 4 out]
      }
      n192 = call "Convert from Dynamic Data"("Dynamic Data Type"=w396) -> ("Array"=w386:dbl[][])  [unwired: 3 in]
      "Config File" <- w386
      n193 = Array Subset(array=w386, index (row)=20 ("index"), length (row)=10 ("length")) -> (w393:dbl[][])  [unwired: 2 in]
      n194 = Array Subset(array=w386, index (row)=10 ("index"), length (row)=10 ("length")) -> (w388:dbl[][])  [unwired: 2 in]
      n195 = Array Subset(array=w386, index (row)=0 ("index"), length (row)=10 ("length")) -> (w387:dbl[][])  [unwired: 2 in]
      n196 = Array Subset(array=w386, index (row)=30 ("index"), length (row)=8 ("length")) -> (w375:dbl[][])  [unwired: 2 in]
      n197 = property on="PumpSeq 4" class="Arr (strict)"("Val(Sgnl)"=w393) -> ()  [unwired: 2 in, 2 out]
      n198 = property on="PumpSeq 2" class="Arr (strict)"("Val(Sgnl)"=w388) -> ()  [unwired: 2 in, 2 out]
      n199 = property on="PumpSeq 3" class="Arr (strict)"("Val(Sgnl)"=w387) -> ()  [unwired: 2 in, 2 out]
      n200 = Index Array(array=w375, index (row)=2, index (col)=0 ("disabled index (col)")) -> ()  [unwired: 1 out]
      n201 = Index Array(array=w375, index (row)=4, index (col)=0 ("disabled index (col)")) -> ()  [unwired: 1 out]
      n202 = Index Array(array=w375, index (row)=0, index (col)=1 ("disabled index (col)")) -> ()  [unwired: 1 out]
      n203 = Index Array(array=w375, index (row)=1, index (col)=1 ("disabled index (col)")) -> ()  [unwired: 1 out]
    }
    n204 = Merge Signals(w163, w164, w23) -> (w58:dynamicdata)
    n205 = call "Build Table"("Include time data"=TRUE, "Signals"=w58) -> ("Table"=w282:string[][])  [unwired: 3 in, 6 out]
    n206 = Delete From Array(array=w282, length=13, index (col)=0 ("index (row)")) -> (array with subset deleted=→"Table":string[][])  [unwired: 1 in, 1 out]
    n207 = Initialize Array(FALSE, 1 ("dimension size")) -> (w13:bool[])
    n208 = And(x="MASTER CONTROL", y="?") -> (x .and. y?=w6:bool)
    n209 = Replace Array Subset(array=w13, new element=w6, index=0) -> (w12:bool[])
    n210 = Index Array(array=w10, index="PORT") -> (element=w9:dbl)
    n211 = call "filenameparser_09.vi"("Description"="Description", "start path"="Browse folder", "Project name"="Project name", "User (initials)"="User (initials)", "OK Button in"="OK Button 2") -> ("appended path 2"=w99:path, "appended path"=w278:path)  [unwired: 4 in, 1 out]
    "Output File" <- w99
    n212 = Boolean To (0,1)(Boolean="OK Button") -> (0, 1=w277:i16)
    n213 = call "Convert to Dynamic Data5"("Double"=w9) -> ("Dynamic Data Type"=→"Waveform Chart 15":dynamicdata)  [unwired: 3 in]
    n214 = for {
      N: w277 -> [_]
      tunnel: w278 -> [w365]
      w369 = " " ("string")
      n215 = property on="Add comment" class="Str"("Val(Sgnl)"="" ("Value (Signaling)")) -> ()  [unwired: 2 in, 2 out]
      n216 = Get Date/Time String(want seconds? (F)=TRUE) -> (date string=w372:string, time string=w370:string)  [unwired: 2 in]
      n217 = Concatenate Strings(w372, w369, w370, w369, "Add comment") -> (w368:string)
      n218 = feedback #8() -> (w367:string[])  [unwired: 1 in]
      n219 = Build Array (concatenate)(w367, w368) -> (w366:string[])
      n220 = feedback-in #8(w366) -> ()
      n221 = Write to Text File(file (use dialog)=w365, text=w366) -> ()  [unwired: 2 in, 3 out]
    }
    n222 = call "DAQ Assistant"("data"=w12, "device name"="device name (PAM)") -> ()  [unwired: 16 in, 2 out]
    n223 = call "Header Names 4.vi"("Dynamic Data"=w58) -> ("Signals Out"=w59:dynamicdata)  [unwired: 10 in]
    n224 = call "Write To Measurement File"("Signals"=w59, "Enable"="OK Button 2", "Filename"=w99) -> ()  [unwired: 14 in, 3 out]
    "Boolean" <- "OK Button 2"
  }
